vi "4155C Report error.vi"(0 "new error":bool, 1 "error message":string, 3 "error in (no error)":errorcluster, 4 "source":string) -> (5 "error out":errorcluster)   [LabVIEW 2016]
doc: "This is a utility VI which reports instrument specific errors when:\n - new error is set to TRUE (ie. there is a new error present)\n - no previous error (no error in \"Error In\" is TRUE).\nso that only the first error occurred will be reported.\n\nThen \n - \"no error\" in \"Error Out\" will be set to \"FALSE\"\n - \"code\" will be set to \"-1300\" - instrument specific error.\n - \"source\" will be set to \"source\" and \"error message\"."
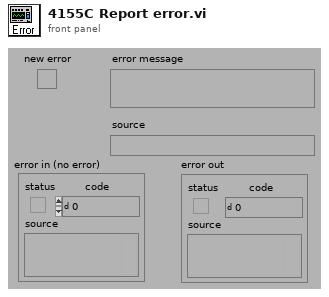
[diagram p1: front panel]
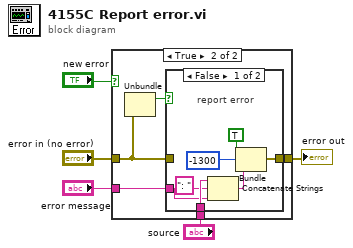
[diagram p0: block diagram]
diagram:
  n1 = case shown="True" "new error" {
    tunnel: [w6 w9] -> w2
    tunnel: "error in (no error)" -> [w6 w10]
    tunnel: "error message" -> [_ w8]
    tunnel: "source" -> [_ w7]
    frame False {
      # "no new error"
    }
    frame True {
      n2 = Unbundle(w10) -> ("status"=w11:bool)  [unwired: 2 out]
      n3 = case shown="False" w11 {
        tunnel: w10 -> [_ w19]
        tunnel: [w16 w19] -> w9
        tunnel: w8 -> [w13 _]
        tunnel: w7 -> [w14 _]
        frame False {
          # "report error"
          n4 = Concatenate Strings(w14, ": ", w13) -> (w15:string)
          n5 = Bundle(TRUE, -1300, w15) -> (w16:errorcluster)  [unwired: 1 in]
        }
        frame True {
          # "previous error\nexisting"
        }
      }
    }
  }
  "error out" <- w2
